vi "Decode Scan Data.vi"(8 "error in (no error)":errorcluster, 10 "Packet Data In":string, 11 "Packet A in":refnum<class "Packet A.lvclass">) -> (0 "error out":errorcluster, 3 "Packet A out":refnum<class "Packet A.lvclass">)   [LabVIEW 2019, in "Packet A.lvclass"]
uses:
  Packet A.lvclass
  Packet A.lvclass/Packet A.ctl
panel:
  out "Magic Byte":u16 format="%x"
  out "length":i32
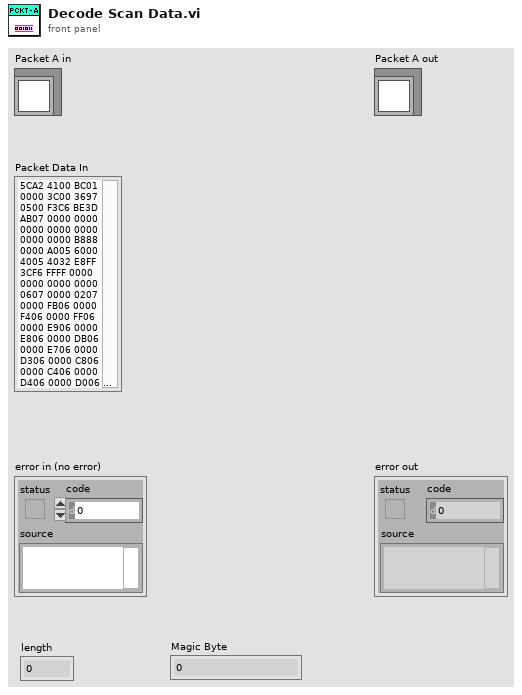
[diagram p1: front panel]
types:
  T1 = enum16{"big-endian, network order", "native, host order", "little-endian"}
  T2 = cluster{"Packet Type":u16, "Packet Size":u32, "Header Size":u16, "Scan Number":u16, "Packet Number":u16, "Timestamp Raw":u64, "Timestamp Sync":u64, "Status Flags":u32, "Scan Frequency":u32, "Num_Points_Scan":u16, "Num_Points_Packet":u16, "First_Index":u16, "First Angle":i32, "Angular Increment":i32, "IQ Input":u32, "IQ Overload":u32}
  T3 = cluster{"Packet Type":u16, "Packet Size":u32, "Header Size":u16, "Scan Number":u16, "Packet Number":u16, "Timestamp Raw":u64, "Timestamp Sync":u64, "Status Flags":u32, "Scan Frequency":u32, "Num_Points_Scan":u16, "Num_Points_Packet":u16, "First_Index":u16, "First Angle":i32, "Angular Increment":i32, "IQ Input":u32, "IQ Overload":u32, "IQ Timestamp Raw":u64, "IQ Timestamp Sync":u64, "Header Padding":u8}
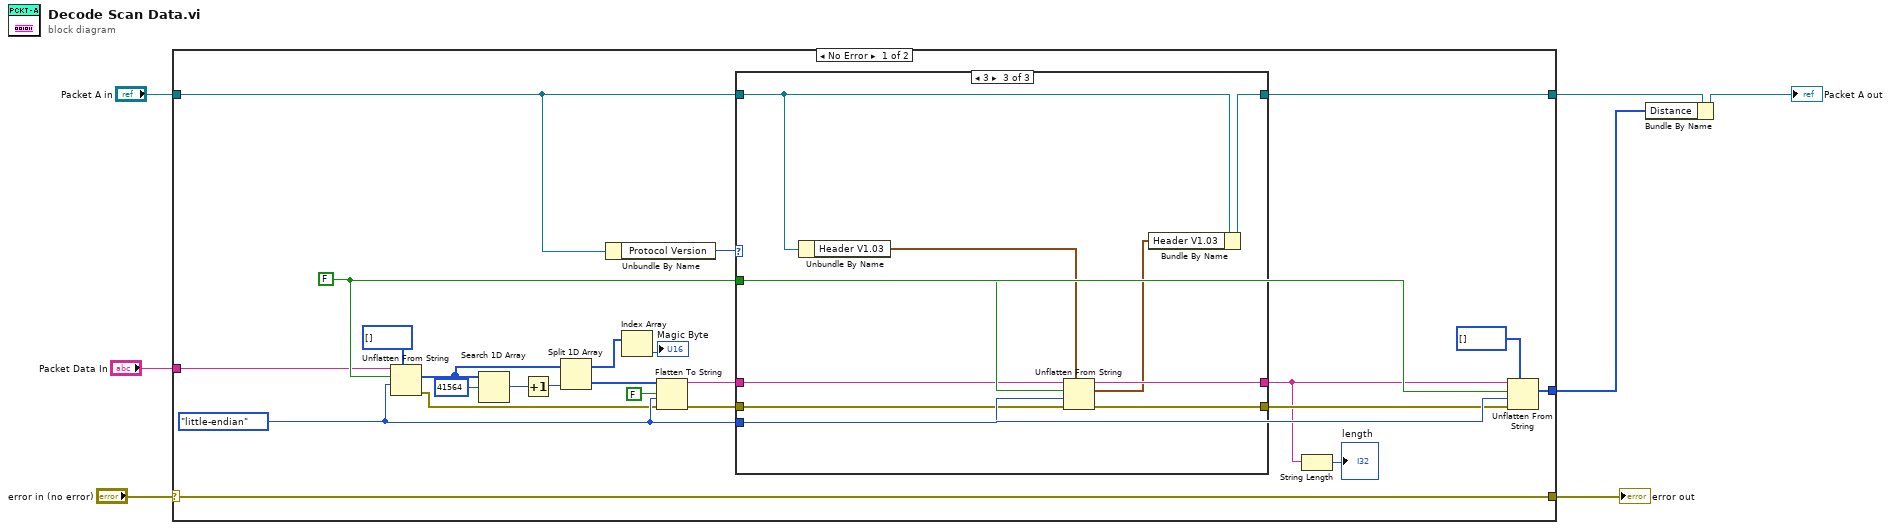
[diagram p0: block diagram]
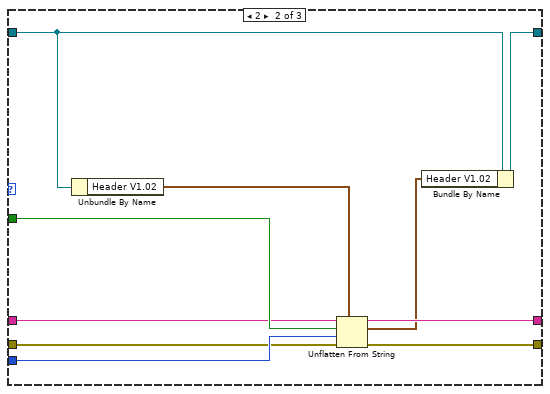
[diagram p3: hidden frame]
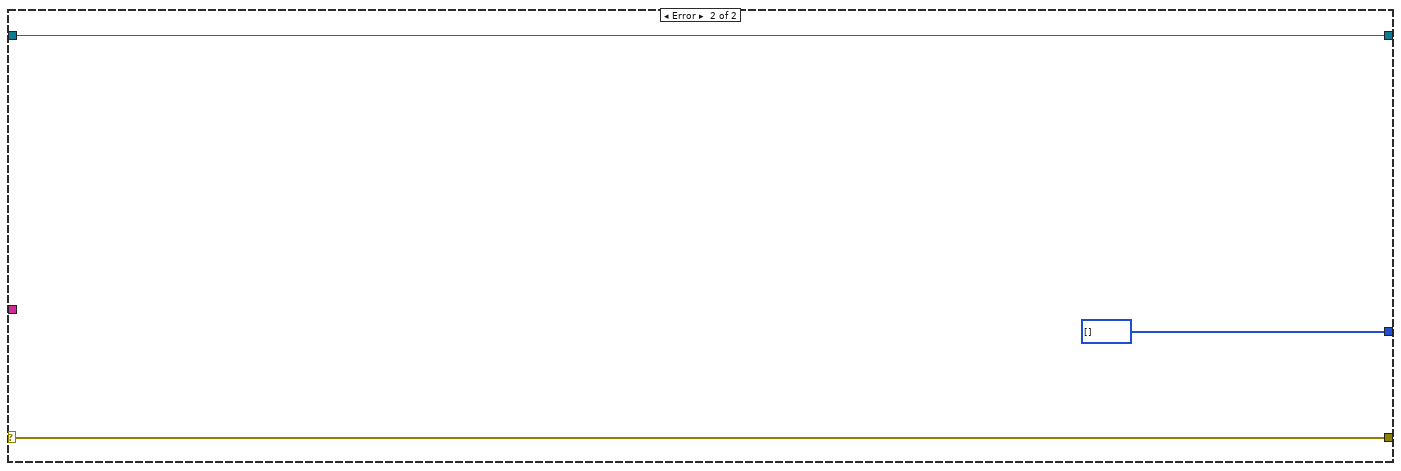
[diagram p4: hidden frame]
diagram:
  n1 = case shown="No Error" "error in (no error)" {
    selector: "error in (no error)" -> [w14 w56]
    tunnel: "Packet Data In" -> [w28 _]
    tunnel: [w26 u32[] []] -> w1
    tunnel: [w14 w56] -> w5
    tunnel: "Packet A in" -> [w9 w55]
    tunnel: [w10 w55] -> w3
    frame No Error {
      w29 = FALSE ("data includes array or string size? (T)")
      w31 = T1."little-endian" ("byte order (0:big-endian, network order)")
      n2 = Unflatten From String(type=u16[] [], binary string=w28, data includes array or string size? (T)=w29, byte order (0:big-endian, network order)=w31) -> (value=w17:u16[], error out=w18:errorcluster)  [unwired: 1 in, 1 out]
      n3 = Search 1D Array(1D array=w17, element=u16 41564) -> (index of element=w24:i32)  [unwired: 1 in]
      n4 = Increment(x=w24) -> (x+1=w25:i32)
      n5 = Split 1D Array(array=w17, index=w25) -> (first subarray=w16:u16[], second subarray=w21:u16[])
      n6 = Unbundle By Name(w9) -> ("Protocol Version"=w8:i32)
      n7 = Index Array(array=w16) -> (element=→"Magic Byte":u16)  [unwired: 1 in]
      n8 = Flatten To String(anything=w21, prepend array or string size? (T)=FALSE, byte order (0:big-endian, network order)=w31, error in (no error)=w18) -> (data string=w13:string, error out=w19:errorcluster)  [unwired: 1 out]
      n9 = case shown="3" w8 {
        tunnel: w31 -> [_ w44 w54]
        tunnel: [w32 w43 w53] -> w30
        tunnel: w29 -> [_ w42 w52]
        tunnel: w19 -> [w32 w41 w51]
        tunnel: w13 -> [w33 w40 w50]
        tunnel: [w33 w39 w49] -> w11
        tunnel: w9 -> [w34 w38 w48]
        tunnel: [w34 w36 w46] -> w10
        frame 0, Default {
        }
        frame 2 {
          n10 = Unbundle By Name(w38) -> ("Header V1.02"=w37:T2)
          n11 = Unflatten From String(type=w37, binary string=w40, data includes array or string size? (T)=w42, byte order (0:big-endian, network order)=w44, error in (no error)=w41) -> (rest of the binary string=w39:string, value=w35:T2, error out=w43:errorcluster)
          n12 = Bundle By Name(cluster=w38, "Header V1.02"=w35) -> (w36:refnum<class "Packet A.lvclass">)
        }
        frame 3 {
          n13 = Unbundle By Name(w48) -> ("Header V1.03"=w47:T3)
          n14 = Unflatten From String(type=w47, binary string=w50, data includes array or string size? (T)=w52, byte order (0:big-endian, network order)=w54, error in (no error)=w51) -> (rest of the binary string=w49:string, value=w45:T3, error out=w53:errorcluster)
          n15 = Bundle By Name(cluster=w48, "Header V1.03"=w45) -> (w46:refnum<class "Packet A.lvclass">)
        }
      }
      n16 = String Length(string=w11) -> (length=→"length":i32)
      n17 = Unflatten From String(type=u32[] [], binary string=w11, data includes array or string size? (T)=w29, byte order (0:big-endian, network order)=w31, error in (no error)=w30) -> (value=w26:u32[])  [unwired: 2 out]
    }
    frame Error {
    }
  }
  "error out" <- w5
  n18 = Bundle By Name(cluster=w3, "Distance"=w1) -> (→"Packet A out":refnum<class "Packet A.lvclass">)
